vi "DSF.Engine.BuilderManager.Create.vi"(7 "number of builders":i32, 8 "error in (no error)":errorcluster, 9 "Framework Cache":refnum<class "DSF.Engine.Memory.Cache.Framework.lvclass">, 10 "Builder type":refnum<class "DSF.Engine.Builder.lvclass">, 11 "Builder Manager type":refnum<class "DSF.Engine.BuilderManager.lvclass">) -> (0 "error out":errorcluster, 3 "Builder Manager":refnum<class "DSF.Engine.BuilderManager.lvclass">)   [LabVIEW 2016, in "DSF.Engine.lvlib" / "DSF.Engine.BuilderManager.lvclass"]
uses:
  DSF.Engine.BuilderManager.lvclass
  Cache/DSF.Engine.Memory.Cache.Framework.lvclass
  Builder/DSF.Engine.Builder.lvclass
  DSF.Engine.BuilderManager.lvclass/DSF.Engine.BuilderManager.ctl
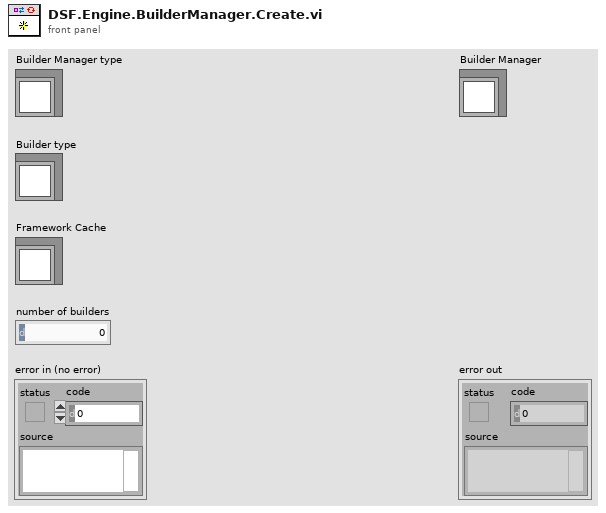
[diagram p1: front panel]
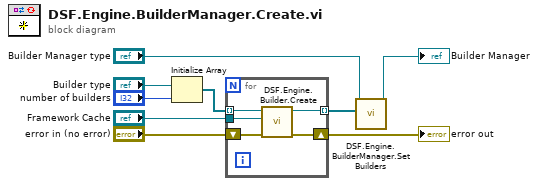
[diagram p0: block diagram]
diagram:
  n1 = Initialize Array("Builder type", "number of builders") -> (w5:refnum<class "DSF.Engine.Builder.lvclass">[])
  n2 = for {
    tunnel: "Framework Cache" -> [w14]
    tunnel: w5 -> [w12] mode=indexing
    tunnel: [w11] -> w4 mode=indexing
    shift-right: [w10] -> w1
    shift-left: "error in (no error)" -> [w13]
    n3 = call "DSF.Engine.Builder.Create.vi"("error in (no error)"=w13, "Framework Cache"=w14, "Builder type"=w12) -> ("error out"=w10:errorcluster, "Builder"=w11:refnum<class "DSF.Engine.Builder.lvclass">)  [unwired: 7 in]
  }
  "error out" <- w1
  n4 = call "DSF.Engine.BuilderManager.Set Builders.vi"("Builders"=w4, "Builder Manager in"="Builder Manager type") -> ("Builder Manager out"=→"Builder Manager":refnum<class "DSF.Engine.BuilderManager.lvclass">)  [unwired: 9 in]
